vi "Create Actions.vi"(0 "Script":T2) -> (4 "Actions out":T1[](array[typedef]))   [LabVIEW 2019]
uses:
  TypeDef/Action.ctl
  TypeDef/ScriptName.ctl
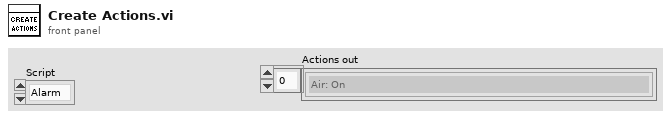
[diagram p1: front panel]
types:
  T1 = typedef "Action.ctl" = enum16{"Air: On", "Air: Off", "Pump Station: On (Filling Mode)", "Pump Station: On (Pressure Mode)", "Pump Station: Off", "Air Valves: Open (DUT Filling)", "Air Valves: Open (Chamber Filling)", "Air Valves: Open (Pump Pressure – DUT)", "Air Valves: Open (Pump Pressure – Chamber)", "Air Valves: Open (Haskel Pressure – DUT)", "Air Valves: Open (Haskel Pressure – Chamber)", "Air Valves: Open (Slow Release – DUT)", "Air Valves: Open (Slow Release – Chamber)", "Air Valves: Open (Fast Release – DUT)", "Air Valves: Open (Fast Release – Chamber)", "Air Valves: Open (Emergency Release – DUT and Chamber)", "Air Valves: Open (Leak Test – Pressure Sensor 41.3)", "Air Valves: Open (Leak Test – Burette 42)", "Air Valves: Fully Closed", "Haskel: Off (0)", "Haskel: Pressure Control (PI Regulator)", "Haskel: Measure T0", "Proportional Valve: Off (0)", "Proportional Valve: Pressure Control (PI Regulator)", "Proportional Valve: Measure T0", "Valve 44.1: Open", "Valve 44.1: Close", "Valve 44.2: Open", "Valve 44.2: Close", "Valve 37.1: Open", "Valve 37.1: Close", "Valve 37.2: Open", "Valve 37.2: Close", "Filling: In Progress", "Pressure pre-loading: DUT", "Pressure pre-loading: Chamber", "Slow Pressure Release: In Progress (DUT)", "Slow Pressure Release: In Progress (Chamber)", "NONE"}
  T2 = typedef "ScriptName.ctl" = enum16{"Alarm", "Filling DUT", "Filling Chamber", "Measure Haskel T0 DUT", "Measure Haskel T0 Chamber", "Measure Pump T0 DUT", "Measure Pump T0 Chamber", "Low Pressure DUT", "Low Pressure Chamber", "Hi Pressure Dut", "Hi Pressure Chamber", "Stop Pump"}
  T3 = typedef "Action.ctl" = enum16{"Air: On", "Air: Off", "Pump Station: On (Filling Mode)", "Pump Station: On (Pressure Mode)", "Pump Station: Off", "Air Valves: Open (DUT Filling)", "Air Valves: Open (Chamber Filling)", "Air Valves: Open (Pump Pressure – DUT)", "Air Valves: Open (Pump Pressure – Chamber)", "Air Valves: Open (Haskel Pressure – DUT)", "Air Valves: Open (Haskel Pressure – Chamber)", "Air Valves: Open (Slow Release – DUT)", "Air Valves: Open (Slow Release – Chamber)", "Air Valves: Open (Fast Release – DUT)", "Air Valves: Open (Fast Release – Chamber)", "Air Valves: Open (Emergency Release – DUT & Chamber)", "Air Valves: Open (Leak Test – Pressure Sensor 41.3)", "Air Valves: Open (Leak Test – Burette 42)", "Air Valves: Fully Closed", "Haskel: Off (0)", "Haskel: Pressure Control (PI Regulator)", "Haskel: Measure T0", "Proportional Valve: Off (0)", "Proportional Valve: Pressure Control (PI Regulator)", "Proportional Valve: Measure T0", "Valve 44.1: Open", "Valve 44.1: Close", "Valve 44.2: Open", "Valve 44.2: Close", "Valve 37.1: Open", "Valve 37.1: Close", "Valve 37.2: Open", "Valve 37.2: Close", "Filling: In Progress", "Pressure pre-loading: DUT", "Pressure pre-loading: Chamber", "Slow Pressure Release: In Progress (DUT)", "Slow Pressure Release: In Progress (Chamber)", "NONE"}
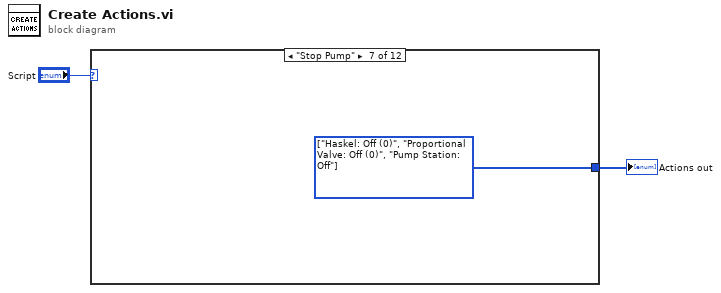
[diagram p0: block diagram]
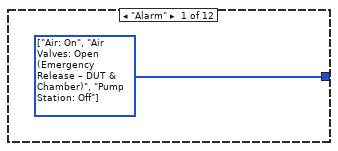
[diagram p2: hidden frame]
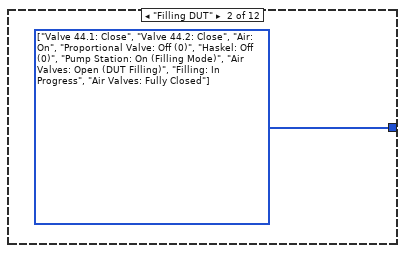
[diagram p3: hidden frame]
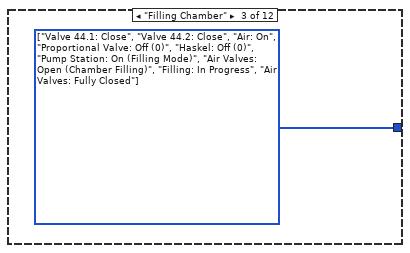
[diagram p4: hidden frame]
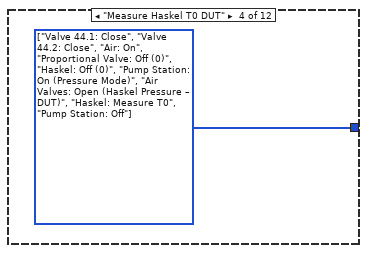
[diagram p5: hidden frame]
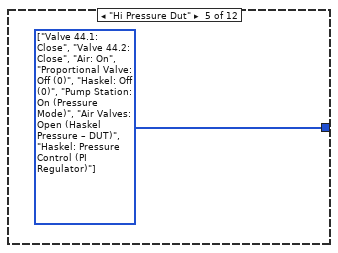
[diagram p6: hidden frame]
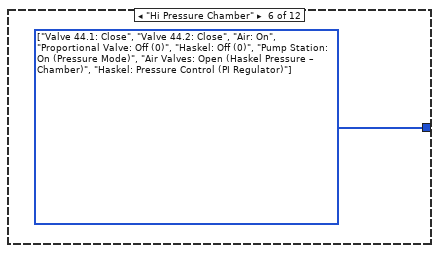
[diagram p7: hidden frame]
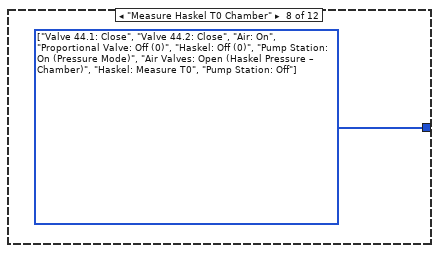
[diagram p8: hidden frame]
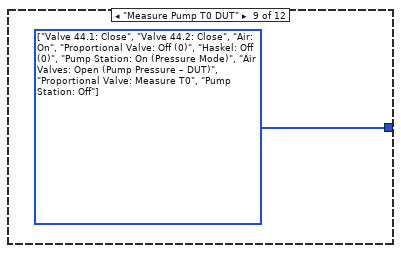
[diagram p9: hidden frame]
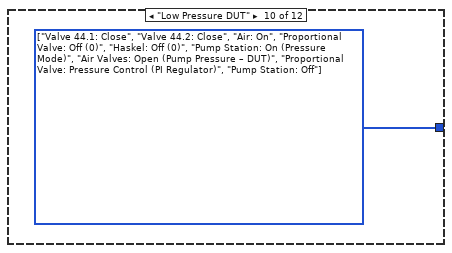
[diagram p10: hidden frame]
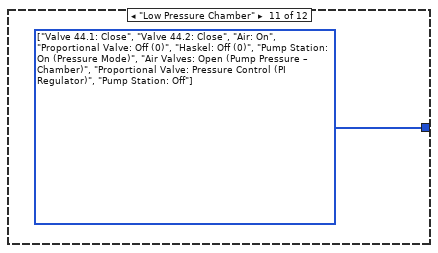
[diagram p11: hidden frame]
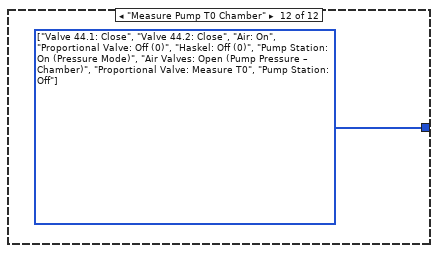
[diagram p12: hidden frame]
diagram:
  n1 = case shown="\"Stop Pump\"" "Script" {
    tunnel: [w3 w4 w5 w6 w7 w8 w9 w10 w11 w12 w13 w14] -> w1
    frame "Alarm" {
      w3 = T3[] [enum."Air: On", enum."Air Valves: Open (Emergency Release – DUT & Chamber)", enum."Pump Station: Off"] items=["Air: On", "Air: Off", "Pump Station: On (Filling Mode)", "Pump Station: On (Pressure Mode)", "Pump Station: Off", "Air Valves: Open (DUT Filling)", "Air Valves: Open (Chamber Filling)", "Air Valves: Open (Pump Pressure – DUT)", "Air Valves: Open (Pump Pressure – Chamber)", "Air Valves: Open (Haskel Pressure – DUT)", "Air Valves: Open (Haskel Pressure – Chamber)", "Air Valves: Open (Slow Release – DUT)", "Air Valves: Open (Slow Release – Chamber)", "Air Valves: Open (Fast Release – DUT)", "Air Valves: Open (Fast Release – Chamber)", "Air Valves: Open (Emergency Release – DUT & Chamber)", "Air Valves: Open (Leak Test – Pressure Sensor 41.3)", "Air Valves: Open (Leak Test – Burette 42)", "Air Valves: Fully Closed", "Haskel: Off (0)", "Haskel: Pressure Control (PI Regulator)", "Haskel: Measure T0", "Proportional Valve: Off (0)", "Proportional Valve: Pressure Control (PI Regulator)", "Proportional Valve: Measure T0", "Valve 44.1: Open", "Valve 44.1: Close", "Valve 44.2: Open", "Valve 44.2: Close", "Valve 37.1: Open", "Valve 37.1: Close", "Valve 37.2: Open", "Valve 37.2: Close", "Filling: In Progress", "Pressure pre-loading: DUT", "Pressure pre-loading: Chamber", "Slow Pressure Release: In Progress (DUT)", "Slow Pressure Release: In Progress (Chamber)", "NONE"] ("Actions")
    }
    frame "Filling DUT" {
      w4 = T1[] [enum."Valve 44.1: Close", enum."Valve 44.2: Close", enum."Air: On", enum."Proportional Valve: Off (0)", enum."Haskel: Off (0)", enum."Pump Station: On (Filling Mode)", enum."Air Valves: Open (DUT Filling)", enum."Filling: In Progress", enum."Air Valves: Fully Closed"] items=["Air: On", "Air: Off", "Pump Station: On (Filling Mode)", "Pump Station: On (Pressure Mode)", "Pump Station: Off", "Air Valves: Open (DUT Filling)", "Air Valves: Open (Chamber Filling)", "Air Valves: Open (Pump Pressure – DUT)", "Air Valves: Open (Pump Pressure – Chamber)", "Air Valves: Open (Haskel Pressure – DUT)", "Air Valves: Open (Haskel Pressure – Chamber)", "Air Valves: Open (Slow Release – DUT)", "Air Valves: Open (Slow Release – Chamber)", "Air Valves: Open (Fast Release – DUT)", "Air Valves: Open (Fast Release – Chamber)", "Air Valves: Open (Emergency Release – DUT and Chamber)", "Air Valves: Open (Leak Test – Pressure Sensor 41.3)", "Air Valves: Open (Leak Test – Burette 42)", "Air Valves: Fully Closed", "Haskel: Off (0)", "Haskel: Pressure Control (PI Regulator)", "Haskel: Measure T0", "Proportional Valve: Off (0)", "Proportional Valve: Pressure Control (PI Regulator)", "Proportional Valve: Measure T0", "Valve 44.1: Open", "Valve 44.1: Close", "Valve 44.2: Open", "Valve 44.2: Close", "Valve 37.1: Open", "Valve 37.1: Close", "Valve 37.2: Open", "Valve 37.2: Close", "Filling: In Progress", "Pressure pre-loading: DUT", "Pressure pre-loading: Chamber", "Slow Pressure Release: In Progress (DUT)", "Slow Pressure Release: In Progress (Chamber)", "NONE"] ("Actions")
    }
    frame "Filling Chamber" {
      w5 = T1[] [enum."Valve 44.1: Close", enum."Valve 44.2: Close", enum."Air: On", enum."Proportional Valve: Off (0)", enum."Haskel: Off (0)", enum."Pump Station: On (Filling Mode)", enum."Air Valves: Open (Chamber Filling)", enum."Filling: In Progress", enum."Air Valves: Fully Closed"] items=["Air: On", "Air: Off", "Pump Station: On (Filling Mode)", "Pump Station: On (Pressure Mode)", "Pump Station: Off", "Air Valves: Open (DUT Filling)", "Air Valves: Open (Chamber Filling)", "Air Valves: Open (Pump Pressure – DUT)", "Air Valves: Open (Pump Pressure – Chamber)", "Air Valves: Open (Haskel Pressure – DUT)", "Air Valves: Open (Haskel Pressure – Chamber)", "Air Valves: Open (Slow Release – DUT)", "Air Valves: Open (Slow Release – Chamber)", "Air Valves: Open (Fast Release – DUT)", "Air Valves: Open (Fast Release – Chamber)", "Air Valves: Open (Emergency Release – DUT and Chamber)", "Air Valves: Open (Leak Test – Pressure Sensor 41.3)", "Air Valves: Open (Leak Test – Burette 42)", "Air Valves: Fully Closed", "Haskel: Off (0)", "Haskel: Pressure Control (PI Regulator)", "Haskel: Measure T0", "Proportional Valve: Off (0)", "Proportional Valve: Pressure Control (PI Regulator)", "Proportional Valve: Measure T0", "Valve 44.1: Open", "Valve 44.1: Close", "Valve 44.2: Open", "Valve 44.2: Close", "Valve 37.1: Open", "Valve 37.1: Close", "Valve 37.2: Open", "Valve 37.2: Close", "Filling: In Progress", "Pressure pre-loading: DUT", "Pressure pre-loading: Chamber", "Slow Pressure Release: In Progress (DUT)", "Slow Pressure Release: In Progress (Chamber)", "NONE"] ("Actions")
    }
    frame "Measure Haskel T0 DUT" {
      w6 = T1[] [enum."Valve 44.1: Close", enum."Valve 44.2: Close", enum."Air: On", enum."Proportional Valve: Off (0)", enum."Haskel: Off (0)", enum."Pump Station: On (Pressure Mode)", enum."Air Valves: Open (Haskel Pressure – DUT)", enum."Haskel: Measure T0", enum."Pump Station: Off"] items=["Air: On", "Air: Off", "Pump Station: On (Filling Mode)", "Pump Station: On (Pressure Mode)", "Pump Station: Off", "Air Valves: Open (DUT Filling)", "Air Valves: Open (Chamber Filling)", "Air Valves: Open (Pump Pressure – DUT)", "Air Valves: Open (Pump Pressure – Chamber)", "Air Valves: Open (Haskel Pressure – DUT)", "Air Valves: Open (Haskel Pressure – Chamber)", "Air Valves: Open (Slow Release – DUT)", "Air Valves: Open (Slow Release – Chamber)", "Air Valves: Open (Fast Release – DUT)", "Air Valves: Open (Fast Release – Chamber)", "Air Valves: Open (Emergency Release – DUT and Chamber)", "Air Valves: Open (Leak Test – Pressure Sensor 41.3)", "Air Valves: Open (Leak Test – Burette 42)", "Air Valves: Fully Closed", "Haskel: Off (0)", "Haskel: Pressure Control (PI Regulator)", "Haskel: Measure T0", "Proportional Valve: Off (0)", "Proportional Valve: Pressure Control (PI Regulator)", "Proportional Valve: Measure T0", "Valve 44.1: Open", "Valve 44.1: Close", "Valve 44.2: Open", "Valve 44.2: Close", "Valve 37.1: Open", "Valve 37.1: Close", "Valve 37.2: Open", "Valve 37.2: Close", "Filling: In Progress", "Pressure pre-loading: DUT", "Pressure pre-loading: Chamber", "Slow Pressure Release: In Progress (DUT)", "Slow Pressure Release: In Progress (Chamber)", "NONE"] ("Actions")
    }
    frame "Hi Pressure Dut" {
      w7 = T1[] [enum."Valve 44.1: Close", enum."Valve 44.2: Close", enum."Air: On", enum."Proportional Valve: Off (0)", enum."Haskel: Off (0)", enum."Pump Station: On (Pressure Mode)", enum."Air Valves: Open (Haskel Pressure – DUT)", enum."Haskel: Pressure Control (PI Regulator)"] items=["Air: On", "Air: Off", "Pump Station: On (Filling Mode)", "Pump Station: On (Pressure Mode)", "Pump Station: Off", "Air Valves: Open (DUT Filling)", "Air Valves: Open (Chamber Filling)", "Air Valves: Open (Pump Pressure – DUT)", "Air Valves: Open (Pump Pressure – Chamber)", "Air Valves: Open (Haskel Pressure – DUT)", "Air Valves: Open (Haskel Pressure – Chamber)", "Air Valves: Open (Slow Release – DUT)", "Air Valves: Open (Slow Release – Chamber)", "Air Valves: Open (Fast Release – DUT)", "Air Valves: Open (Fast Release – Chamber)", "Air Valves: Open (Emergency Release – DUT and Chamber)", "Air Valves: Open (Leak Test – Pressure Sensor 41.3)", "Air Valves: Open (Leak Test – Burette 42)", "Air Valves: Fully Closed", "Haskel: Off (0)", "Haskel: Pressure Control (PI Regulator)", "Haskel: Measure T0", "Proportional Valve: Off (0)", "Proportional Valve: Pressure Control (PI Regulator)", "Proportional Valve: Measure T0", "Valve 44.1: Open", "Valve 44.1: Close", "Valve 44.2: Open", "Valve 44.2: Close", "Valve 37.1: Open", "Valve 37.1: Close", "Valve 37.2: Open", "Valve 37.2: Close", "Filling: In Progress", "Pressure pre-loading: DUT", "Pressure pre-loading: Chamber", "Slow Pressure Release: In Progress (DUT)", "Slow Pressure Release: In Progress (Chamber)", "NONE"] ("Actions")
    }
    frame "Hi Pressure Chamber" {
      w8 = T1[] [enum."Valve 44.1: Close", enum."Valve 44.2: Close", enum."Air: On", enum."Proportional Valve: Off (0)", enum."Haskel: Off (0)", enum."Pump Station: On (Pressure Mode)", enum."Air Valves: Open (Haskel Pressure – Chamber)", enum."Haskel: Pressure Control (PI Regulator)"] items=["Air: On", "Air: Off", "Pump Station: On (Filling Mode)", "Pump Station: On (Pressure Mode)", "Pump Station: Off", "Air Valves: Open (DUT Filling)", "Air Valves: Open (Chamber Filling)", "Air Valves: Open (Pump Pressure – DUT)", "Air Valves: Open (Pump Pressure – Chamber)", "Air Valves: Open (Haskel Pressure – DUT)", "Air Valves: Open (Haskel Pressure – Chamber)", "Air Valves: Open (Slow Release – DUT)", "Air Valves: Open (Slow Release – Chamber)", "Air Valves: Open (Fast Release – DUT)", "Air Valves: Open (Fast Release – Chamber)", "Air Valves: Open (Emergency Release – DUT and Chamber)", "Air Valves: Open (Leak Test – Pressure Sensor 41.3)", "Air Valves: Open (Leak Test – Burette 42)", "Air Valves: Fully Closed", "Haskel: Off (0)", "Haskel: Pressure Control (PI Regulator)", "Haskel: Measure T0", "Proportional Valve: Off (0)", "Proportional Valve: Pressure Control (PI Regulator)", "Proportional Valve: Measure T0", "Valve 44.1: Open", "Valve 44.1: Close", "Valve 44.2: Open", "Valve 44.2: Close", "Valve 37.1: Open", "Valve 37.1: Close", "Valve 37.2: Open", "Valve 37.2: Close", "Filling: In Progress", "Pressure pre-loading: DUT", "Pressure pre-loading: Chamber", "Slow Pressure Release: In Progress (DUT)", "Slow Pressure Release: In Progress (Chamber)", "NONE"] ("Actions")
    }
    frame "Stop Pump" {
      w9 = T1[] [enum."Haskel: Off (0)", enum."Proportional Valve: Off (0)", enum."Pump Station: Off"] items=["Air: On", "Air: Off", "Pump Station: On (Filling Mode)", "Pump Station: On (Pressure Mode)", "Pump Station: Off", "Air Valves: Open (DUT Filling)", "Air Valves: Open (Chamber Filling)", "Air Valves: Open (Pump Pressure – DUT)", "Air Valves: Open (Pump Pressure – Chamber)", "Air Valves: Open (Haskel Pressure – DUT)", "Air Valves: Open (Haskel Pressure – Chamber)", "Air Valves: Open (Slow Release – DUT)", "Air Valves: Open (Slow Release – Chamber)", "Air Valves: Open (Fast Release – DUT)", "Air Valves: Open (Fast Release – Chamber)", "Air Valves: Open (Emergency Release – DUT and Chamber)", "Air Valves: Open (Leak Test – Pressure Sensor 41.3)", "Air Valves: Open (Leak Test – Burette 42)", "Air Valves: Fully Closed", "Haskel: Off (0)", "Haskel: Pressure Control (PI Regulator)", "Haskel: Measure T0", "Proportional Valve: Off (0)", "Proportional Valve: Pressure Control (PI Regulator)", "Proportional Valve: Measure T0", "Valve 44.1: Open", "Valve 44.1: Close", "Valve 44.2: Open", "Valve 44.2: Close", "Valve 37.1: Open", "Valve 37.1: Close", "Valve 37.2: Open", "Valve 37.2: Close", "Filling: In Progress", "Pressure pre-loading: DUT", "Pressure pre-loading: Chamber", "Slow Pressure Release: In Progress (DUT)", "Slow Pressure Release: In Progress (Chamber)", "NONE"] ("Actions")
    }
    frame "Measure Haskel T0 Chamber" {
      w10 = T1[] [enum."Valve 44.1: Close", enum."Valve 44.2: Close", enum."Air: On", enum."Proportional Valve: Off (0)", enum."Haskel: Off (0)", enum."Pump Station: On (Pressure Mode)", enum."Air Valves: Open (Haskel Pressure – Chamber)", enum."Haskel: Measure T0", enum."Pump Station: Off"] items=["Air: On", "Air: Off", "Pump Station: On (Filling Mode)", "Pump Station: On (Pressure Mode)", "Pump Station: Off", "Air Valves: Open (DUT Filling)", "Air Valves: Open (Chamber Filling)", "Air Valves: Open (Pump Pressure – DUT)", "Air Valves: Open (Pump Pressure – Chamber)", "Air Valves: Open (Haskel Pressure – DUT)", "Air Valves: Open (Haskel Pressure – Chamber)", "Air Valves: Open (Slow Release – DUT)", "Air Valves: Open (Slow Release – Chamber)", "Air Valves: Open (Fast Release – DUT)", "Air Valves: Open (Fast Release – Chamber)", "Air Valves: Open (Emergency Release – DUT and Chamber)", "Air Valves: Open (Leak Test – Pressure Sensor 41.3)", "Air Valves: Open (Leak Test – Burette 42)", "Air Valves: Fully Closed", "Haskel: Off (0)", "Haskel: Pressure Control (PI Regulator)", "Haskel: Measure T0", "Proportional Valve: Off (0)", "Proportional Valve: Pressure Control (PI Regulator)", "Proportional Valve: Measure T0", "Valve 44.1: Open", "Valve 44.1: Close", "Valve 44.2: Open", "Valve 44.2: Close", "Valve 37.1: Open", "Valve 37.1: Close", "Valve 37.2: Open", "Valve 37.2: Close", "Filling: In Progress", "Pressure pre-loading: DUT", "Pressure pre-loading: Chamber", "Slow Pressure Release: In Progress (DUT)", "Slow Pressure Release: In Progress (Chamber)", "NONE"] ("Actions")
    }
    frame "Measure Pump T0 DUT" {
      w11 = T1[] [enum."Valve 44.1: Close", enum."Valve 44.2: Close", enum."Air: On", enum."Proportional Valve: Off (0)", enum."Haskel: Off (0)", enum."Pump Station: On (Pressure Mode)", enum."Air Valves: Open (Pump Pressure – DUT)", enum."Proportional Valve: Measure T0", enum."Pump Station: Off"] items=["Air: On", "Air: Off", "Pump Station: On (Filling Mode)", "Pump Station: On (Pressure Mode)", "Pump Station: Off", "Air Valves: Open (DUT Filling)", "Air Valves: Open (Chamber Filling)", "Air Valves: Open (Pump Pressure – DUT)", "Air Valves: Open (Pump Pressure – Chamber)", "Air Valves: Open (Haskel Pressure – DUT)", "Air Valves: Open (Haskel Pressure – Chamber)", "Air Valves: Open (Slow Release – DUT)", "Air Valves: Open (Slow Release – Chamber)", "Air Valves: Open (Fast Release – DUT)", "Air Valves: Open (Fast Release – Chamber)", "Air Valves: Open (Emergency Release – DUT and Chamber)", "Air Valves: Open (Leak Test – Pressure Sensor 41.3)", "Air Valves: Open (Leak Test – Burette 42)", "Air Valves: Fully Closed", "Haskel: Off (0)", "Haskel: Pressure Control (PI Regulator)", "Haskel: Measure T0", "Proportional Valve: Off (0)", "Proportional Valve: Pressure Control (PI Regulator)", "Proportional Valve: Measure T0", "Valve 44.1: Open", "Valve 44.1: Close", "Valve 44.2: Open", "Valve 44.2: Close", "Valve 37.1: Open", "Valve 37.1: Close", "Valve 37.2: Open", "Valve 37.2: Close", "Filling: In Progress", "Pressure pre-loading: DUT", "Pressure pre-loading: Chamber", "Slow Pressure Release: In Progress (DUT)", "Slow Pressure Release: In Progress (Chamber)", "NONE"] ("Actions")
    }
    frame "Low Pressure DUT" {
      w12 = T1[] [enum."Valve 44.1: Close", enum."Valve 44.2: Close", enum."Air: On", enum."Proportional Valve: Off (0)", enum."Haskel: Off (0)", enum."Pump Station: On (Pressure Mode)", enum."Air Valves: Open (Pump Pressure – DUT)", enum."Proportional Valve: Pressure Control (PI Regulator)", enum."Pump Station: Off"] items=["Air: On", "Air: Off", "Pump Station: On (Filling Mode)", "Pump Station: On (Pressure Mode)", "Pump Station: Off", "Air Valves: Open (DUT Filling)", "Air Valves: Open (Chamber Filling)", "Air Valves: Open (Pump Pressure – DUT)", "Air Valves: Open (Pump Pressure – Chamber)", "Air Valves: Open (Haskel Pressure – DUT)", "Air Valves: Open (Haskel Pressure – Chamber)", "Air Valves: Open (Slow Release – DUT)", "Air Valves: Open (Slow Release – Chamber)", "Air Valves: Open (Fast Release – DUT)", "Air Valves: Open (Fast Release – Chamber)", "Air Valves: Open (Emergency Release – DUT and Chamber)", "Air Valves: Open (Leak Test – Pressure Sensor 41.3)", "Air Valves: Open (Leak Test – Burette 42)", "Air Valves: Fully Closed", "Haskel: Off (0)", "Haskel: Pressure Control (PI Regulator)", "Haskel: Measure T0", "Proportional Valve: Off (0)", "Proportional Valve: Pressure Control (PI Regulator)", "Proportional Valve: Measure T0", "Valve 44.1: Open", "Valve 44.1: Close", "Valve 44.2: Open", "Valve 44.2: Close", "Valve 37.1: Open", "Valve 37.1: Close", "Valve 37.2: Open", "Valve 37.2: Close", "Filling: In Progress", "Pressure pre-loading: DUT", "Pressure pre-loading: Chamber", "Slow Pressure Release: In Progress (DUT)", "Slow Pressure Release: In Progress (Chamber)", "NONE"] ("Actions")
    }
    frame "Low Pressure Chamber" {
      w13 = T1[] [enum."Valve 44.1: Close", enum."Valve 44.2: Close", enum."Air: On", enum."Proportional Valve: Off (0)", enum."Haskel: Off (0)", enum."Pump Station: On (Pressure Mode)", enum."Air Valves: Open (Pump Pressure – Chamber)", enum."Proportional Valve: Pressure Control (PI Regulator)", enum."Pump Station: Off"] items=["Air: On", "Air: Off", "Pump Station: On (Filling Mode)", "Pump Station: On (Pressure Mode)", "Pump Station: Off", "Air Valves: Open (DUT Filling)", "Air Valves: Open (Chamber Filling)", "Air Valves: Open (Pump Pressure – DUT)", "Air Valves: Open (Pump Pressure – Chamber)", "Air Valves: Open (Haskel Pressure – DUT)", "Air Valves: Open (Haskel Pressure – Chamber)", "Air Valves: Open (Slow Release – DUT)", "Air Valves: Open (Slow Release – Chamber)", "Air Valves: Open (Fast Release – DUT)", "Air Valves: Open (Fast Release – Chamber)", "Air Valves: Open (Emergency Release – DUT and Chamber)", "Air Valves: Open (Leak Test – Pressure Sensor 41.3)", "Air Valves: Open (Leak Test – Burette 42)", "Air Valves: Fully Closed", "Haskel: Off (0)", "Haskel: Pressure Control (PI Regulator)", "Haskel: Measure T0", "Proportional Valve: Off (0)", "Proportional Valve: Pressure Control (PI Regulator)", "Proportional Valve: Measure T0", "Valve 44.1: Open", "Valve 44.1: Close", "Valve 44.2: Open", "Valve 44.2: Close", "Valve 37.1: Open", "Valve 37.1: Close", "Valve 37.2: Open", "Valve 37.2: Close", "Filling: In Progress", "Pressure pre-loading: DUT", "Pressure pre-loading: Chamber", "Slow Pressure Release: In Progress (DUT)", "Slow Pressure Release: In Progress (Chamber)", "NONE"] ("Actions")
    }
    frame "Measure Pump T0 Chamber" {
      w14 = T1[] [enum."Valve 44.1: Close", enum."Valve 44.2: Close", enum."Air: On", enum."Proportional Valve: Off (0)", enum."Haskel: Off (0)", enum."Pump Station: On (Pressure Mode)", enum."Air Valves: Open (Pump Pressure – Chamber)", enum."Proportional Valve: Measure T0", enum."Pump Station: Off"] items=["Air: On", "Air: Off", "Pump Station: On (Filling Mode)", "Pump Station: On (Pressure Mode)", "Pump Station: Off", "Air Valves: Open (DUT Filling)", "Air Valves: Open (Chamber Filling)", "Air Valves: Open (Pump Pressure – DUT)", "Air Valves: Open (Pump Pressure – Chamber)", "Air Valves: Open (Haskel Pressure – DUT)", "Air Valves: Open (Haskel Pressure – Chamber)", "Air Valves: Open (Slow Release – DUT)", "Air Valves: Open (Slow Release – Chamber)", "Air Valves: Open (Fast Release – DUT)", "Air Valves: Open (Fast Release – Chamber)", "Air Valves: Open (Emergency Release – DUT and Chamber)", "Air Valves: Open (Leak Test – Pressure Sensor 41.3)", "Air Valves: Open (Leak Test – Burette 42)", "Air Valves: Fully Closed", "Haskel: Off (0)", "Haskel: Pressure Control (PI Regulator)", "Haskel: Measure T0", "Proportional Valve: Off (0)", "Proportional Valve: Pressure Control (PI Regulator)", "Proportional Valve: Measure T0", "Valve 44.1: Open", "Valve 44.1: Close", "Valve 44.2: Open", "Valve 44.2: Close", "Valve 37.1: Open", "Valve 37.1: Close", "Valve 37.2: Open", "Valve 37.2: Close", "Filling: In Progress", "Pressure pre-loading: DUT", "Pressure pre-loading: Chamber", "Slow Pressure Release: In Progress (DUT)", "Slow Pressure Release: In Progress (Chamber)", "NONE"] ("Actions")
    }
  }
  "Actions out" <- w1
